vi "Check CDO Channel Settings.vi"(8 "error in":errorcluster, 9 "read channel settings":T1[](array[typedef])=[{"name"="", "default value"=TRUE, "counter driven state"=enum."Disabled"}, {"name"="", "default value"=TRUE, "counter driven state"=enum."Disabled"}, {"name"="", "default value"=TRUE, "counter driven state"=enum."Enabled"}, {"name"="", "default value"=TRUE, "counter driven state"=enum."Disabled"}, {"name"="", "default value"=TRUE, "counter driven state"=enum."Disabled"}, {"name"="", "default value"=TRUE, "counter driven state"=enum."Enabled"}, {"name"="", "default value"=FALSE, "counter driven state"=enum."Enabled"}, {"name"="", "default value"=FALSE, "counter driven state"=enum."Disabled"}], 10 "initial channel settings":T1[](array[typedef])=[{"name"="", "default value"=TRUE, "counter driven state"=enum."Disabled"}, {"name"="", "default value"=TRUE, "counter driven state"=enum."Disabled"}, {"name"="", "default value"=TRUE, "counter driven state"=enum."Enabled"}, {"name"="", "default value"=TRUE, "counter driven state"=enum."Disabled"}, {"name"="", "default value"=TRUE, "counter driven state"=enum."Disabled"}, {"name"="", "default value"=TRUE, "counter driven state"=enum."Enabled"}, {"name"="", "default value"=FALSE, "counter driven state"=enum."Enabled"}, {"name"="", "default value"=FALSE, "counter driven state"=enum."Disabled"}], 11 "TestCase in":refnum<class "TestCase.lvclass">) -> (0 "error out":errorcluster, 3 "TestCase out":refnum<class "TestCase.lvclass">)   [LabVIEW 2017, in "Module Test.lvclass"]
uses:
  Module Test Classes/Module Test.lvclass
  <vilib>/addons/_JKI Toolkits/VI Tester/TestCase.llb/TestCase.lvclass
  Scripting/Modules/Mode Classes/Controls/counter driven output channel settings.ctl
  Scripting/Modules/Channel Classes/Counter Driven Output Channel/Counter Driven State.ctl
  Scripting/Modules/Channel Classes/Counter Driven Output Channel/Counter Driven Output Channel.lvclass
  Scripting/Scan Engine Scripting.lvlib
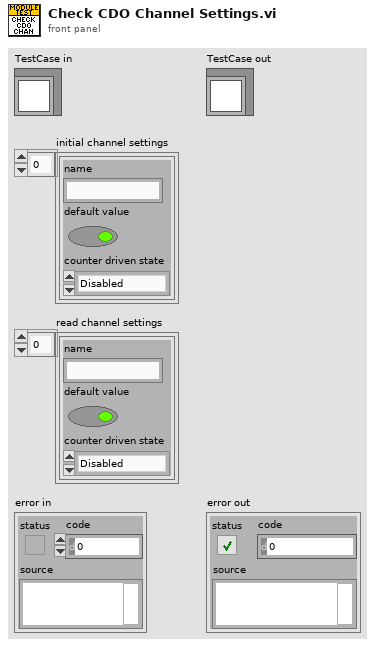
[diagram p1: front panel]
types:
  T1 = typedef "Scan Engine Scripting.lvlib/counter driven output channel settings.ctl" = cluster{"name":string, "default value":bool, "counter driven state":T2}
  T2 = typedef "Scan Engine Scripting.lvlib/Counter Driven Output Channel.lvclass/Counter Driven State.ctl" = enum16{"Disabled", "Enabled"}
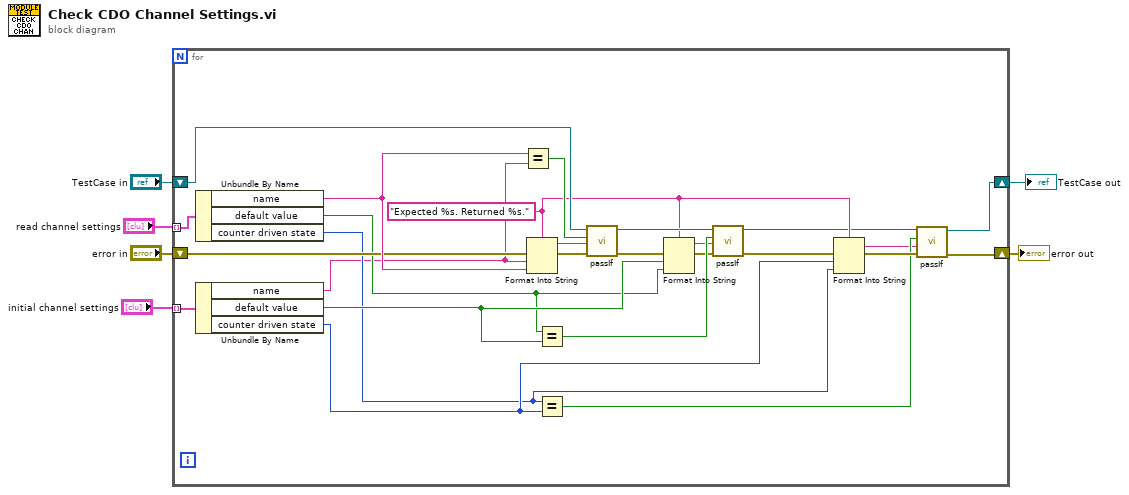
[diagram p0: block diagram]
diagram:
  n1 = for {
    tunnel: "read channel settings" -> [w31] mode=indexing
    tunnel: "initial channel settings" -> [w32] mode=indexing
    shift-right: [w10] -> w5
    shift-left: "TestCase in" -> [w30]
    shift-right: [w8] -> w3
    shift-left: "error in" -> [w26]
    w13 = "Expected %s. Returned %s." ("format string")
    n2 = Unbundle By Name(w31) -> ("name"=w28:string, "default value"=w21:bool, "counter driven state"=w16:T2)
    n3 = Unbundle By Name(w32) -> ("name"=w7:string, "default value"=w22:bool, "counter driven state"=w17:T2)
    n4 = Equal?(x=w28, y=w7) -> (x = y?=w29:bool)
    n5 = Format Into String(format string=w13, error in=w26, w7, w28) -> (resulting string=w27:string, error out=w25:errorcluster)  [unwired: 1 in]
    n6 = Equal?(x=w21, y=w22) -> (x = y?=w23:bool)
    n7 = Equal?(x=w16, y=w17) -> (x = y?=w12:bool)
    n8 = call-dynamic "passIf.vi"("error in (no error)"=w25, "message (\"\")"=w27, "pass"=w29, "TestCase in"=w30) -> ("error out"=w20:errorcluster, "TestCase out"=w24:refnum<class "TestCase.lvclass">)  [unwired: 6 in]
    n9 = Format Into String(format string=w13, error in=w20, w22, w21) -> (resulting string=w18:string, error out=w19:errorcluster)  [unwired: 1 in]
    n10 = call-dynamic "passIf.vi"("error in (no error)"=w19, "message (\"\")"=w18, "pass"=w23, "TestCase in"=w24) -> ("error out"=w15:errorcluster, "TestCase out"=w11:refnum<class "TestCase.lvclass">)  [unwired: 6 in]
    n11 = Format Into String(format string=w13, error in=w15, w17, w16) -> (resulting string=w9:string, error out=w14:errorcluster)  [unwired: 1 in]
    n12 = call-dynamic "passIf.vi"("error in (no error)"=w14, "message (\"\")"=w9, "pass"=w12, "TestCase in"=w11) -> ("error out"=w8:errorcluster, "TestCase out"=w10:refnum<class "TestCase.lvclass">)  [unwired: 6 in]
  }
  "TestCase out" <- w5
  "error out" <- w3
